vi "Launcher (Top Level).vi"   [LabVIEW 2020]
uses:
  Architecture Support/Architecture Support.lvlib
  Main Modules/Controller/Controller.lvlib
  Main Modules/UI/UI.lvlib
  Main Modules/Error Handler/Error Handler.lvlib
  Main Modules/Wait/Wait.lvlib
panel:
  # "NetScan"
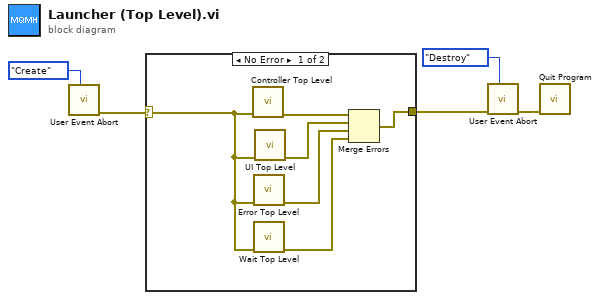
[diagram p0: block diagram]
diagram:
  n1 = call "User Event Abort.vi"("Enum"=enum16{"Create", "Destroy", "Get"}."Create") -> ("error out"=w5:errorcluster)  [unwired: 9 in, 1 out]
  n2 = case shown="No Error" w5 {
    selector: w5 -> [w7 w12]
    tunnel: [w11 w12] -> w1
    frame No Error {
      n3 = call "Controller Top Level.vi"("error in (no error)"=w7) -> ("error out"=w10:errorcluster)  [unwired: 10 in]
      n4 = call "Error Top Level.vi"("error in (no error)"=w7) -> ("error out"=w8:errorcluster)  [unwired: 10 in]
      n5 = call "Wait Top Level.vi"("error in (no error)"=w7) -> ("error out"=w6:errorcluster)  [unwired: 10 in]
      n6 = call "UI Top Level.vi"("error in"=w7) -> ("error out"=w9:errorcluster)  [unwired: 10 in]
      n7 = Merge Errors(w10, w9, w8, w6) -> (w11:errorcluster)
    }
    frame Error {
    }
  }
  n8 = call "User Event Abort.vi"("Enum"=enum16{"Create", "Destroy", "Get"}."Destroy", "error in (no error)"=w1) -> ("error out"=w2:errorcluster)  [unwired: 8 in, 1 out]
  n9 = call "Quit Program.vi"("error in (no error)"=w2) -> ()  [unwired: 11 in]
